vi "Configure Bursted Generation.vi"(0 "RFSG handle":refnum<k15>, 5 "Waveform":T1={"Waveform Name"="Wfm", "Waveform"={"x0"=0.0, "dx"=0.0, "y"=[]}, "Signal Bandwidth (Hz)"=0.0, "PAPR (dB)"=0.0, "Burst Length (s)"=0.0, "Sample Rate"=0.0, "Burst Start Locations"=[], "Burst Stop Locations"=[], "Idle Duration Present?"=FALSE, "Runtime Scaling"=0.0, "Script"=""} {"Runtime Scaling" format="%#_6p"; "Sample Rate" format="%#_6p"; "Burst Length (s)" format="%#_6p"; "PAPR (dB)" format="%.2f"; "Signal Bandwidth (Hz)" format="%#_6p"; "Waveform"."y" format="%.2f"; "Waveform"."dx" format="%^.2e"; "Waveform"."x0" format="%^.2e"}, 7 "Waveform Timing Configuration":T4={"Duty Cycle (%)"=50.0, "Pre-Burst Time (s)"=1e-06, "Post-Burst Time (s)"=1e-06, "Burst Start Trigger Export"="PXI_Trig0"} {"Post-Burst Time (s)" format="%#_6p"; "Pre-Burst Time (s)" format="%#_6p"; "Duty Cycle (%)" min=1.0 max=100.0 step=1.0 format="%#_2d%%"}, 9 "PAEN Configuration":T2={"PAEN Mode"=enum."Dynamic", "PA Enable Trigger Export Terminal"="PFI0", "PA Enable Trigger Mode"=23001, "Command Enable Time (s)"=0.0, "Command Disable Time (s)"=0.0} {"PA Enable Trigger Mode" items=["Pulse"=23000, "Toggle"=23001]; "Command Disable Time (s)" format="%#_6p"; "Command Enable Time (s)" format="%#_6p"}, 11 "error in":errorcluster) -> (4 "RFSG handle out":refnum<k15>, 6 "Waveform out":T1={"Waveform Name"="Wfm", "Waveform"={"x0"=0.0, "dx"=0.0, "y"=[]}, "Signal Bandwidth (Hz)"=0.0, "PAPR (dB)"=0.0, "Burst Length (s)"=0.0, "Sample Rate"=0.0, "Burst Start Locations"=[], "Burst Stop Locations"=[], "Idle Duration Present?"=FALSE, "Runtime Scaling"=0.0, "Script"=""} {"Runtime Scaling" format="%#_6p"; "Sample Rate" format="%#_6p"; "Burst Length (s)" format="%#_6p"; "PAPR (dB)" format="%.2f"; "Signal Bandwidth (Hz)" format="%#_6p"; "Waveform"."y" format="%.2f"; "Waveform"."dx" format="%^.2e"; "Waveform"."x0" format="%^.2e"}, 8 "Generation Period (s)":dbl format="%#_6p", 15 "error out":errorcluster)   [LabVIEW 2016, in "SG.lvlib"]
uses:
  SG.lvlib
  Typedefs/Waveform.ctl
  Typedefs/Waveform Timing Configuration.ctl
  <instrlib>/niRFSG/niRFSG.llb/niRFSG Exported Signal Destinations.ctl
  Typedefs/PAEN Configuration.ctl
  <instrlib>/niRFSG/niRFSG.llb/niRFSG Signal Names.ctl
  <instrlib>/niRFSG/niRFSG.llb/niRFSG Signal Identifiers.ctl
  <instrlib>/niRFSG/niRFSG.llb/niRFSG Script Trigger IDs.ctl
  <instrlib>/niRFSG/niRFSG.llb/niRFSG Configure Script Trigger Software.vi
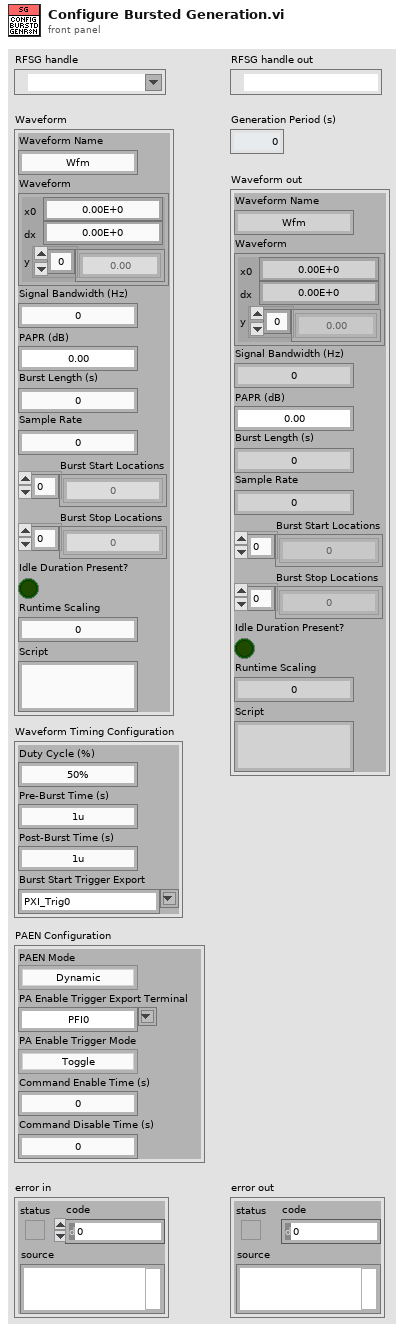
[diagram p1: front panel]
types:
  T1 = typedef "SG.lvlib/Waveform.ctl" = cluster{"Waveform Name":string, "Waveform":cluster{"x0":dbl, "dx":dbl, "y":csg[]}, "Signal Bandwidth (Hz)":dbl, "PAPR (dB)":dbl, "Burst Length (s)":dbl, "Sample Rate":dbl, "Burst Start Locations":i32[], "Burst Stop Locations":i32[], "Idle Duration Present?":bool, "Runtime Scaling":dbl, "Script":string}
  T2 = typedef "SG.lvlib/PAEN Configuration.ctl" = cluster{"PAEN Mode":enum16{"Disabled", "Static", "Dynamic"}, "PA Enable Trigger Export Terminal":T3, "PA Enable Trigger Mode":i32, "Command Enable Time (s)":dbl, "Command Disable Time (s)":dbl}
  T3 = typedef "niRFSG Exported Signal Destinations.ctl" = string
  T4 = typedef "SG.lvlib/Waveform Timing Configuration.ctl" = cluster{"Duty Cycle (%)":dbl, "Pre-Burst Time (s)":dbl, "Post-Burst Time (s)":dbl, "Burst Start Trigger Export":T3}
  T5 = typedef "niRFSG Script Trigger IDs.ctl" = string
  T6 = typedef "niRFSG Signal Identifiers.ctl" = string
  T7 = typedef "niRFSG Signal Names.ctl" = i32
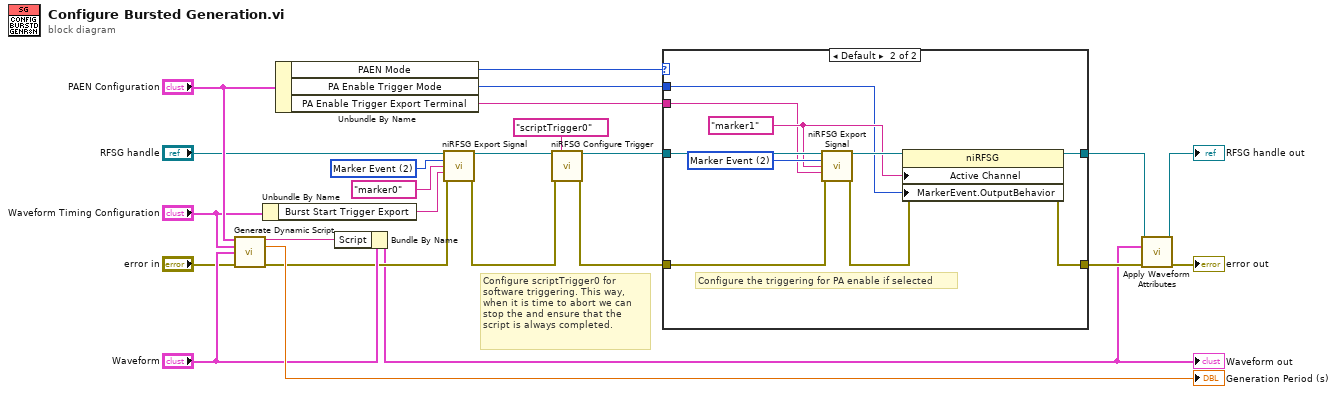
[diagram p0: block diagram]
diagram:
  w17 = T7 2 items=["Start Trigger", "Script Trigger", "Marker Event", "Ref Clock", "Started Event", "Done Event", "Configuration List Step Trigger", "Configuration Settled Event"] ("signal")
  # "Configure scriptTrigger0 for software triggering. This way, when it is time to abort we can stop the and ensure that the script is always completed."
  n1 = call "Generate Dynamic Script.vi"("PAEN Config"="PAEN Configuration", "Waveform Timing Configuration"="Waveform Timing Configuration", "Waveform"="Waveform", "error in (no error)"="error in") -> ("Script"=w8:string, "Generation Period (s)"=→"Generation Period (s)":dbl, "error out"=w6:errorcluster)  [unwired: 9 in]
  n2 = Unbundle By Name("Waveform Timing Configuration") -> ("Burst Start Trigger Export"=w14:T3)
  n3 = Unbundle By Name("PAEN Configuration") -> ("PAEN Mode"=w21:enum16{"Disabled", "Static", "Dynamic"}, "PA Enable Trigger Mode"=w20:i32, "PA Enable Trigger Export Terminal"=w18:T3)
  n4 = Bundle By Name(cluster="Waveform", "Script"=w8) -> (w1:T1)
  "Waveform out" <- w1
  n5 = call <instrlib>:"niRFSG Export Signal.vi"("instrument handle"="RFSG handle", "signal"=w17, "signal identifier"=T6 "marker0", "output terminal"=w14, "error in"=w6) -> ("instrument handle out"=w12:refnum<k15>, "error out"=w11:errorcluster)  [unwired: 9 in]
  n6 = call-poly <instrlib>:"niRFSG Configure Trigger.vi"("instrument handle"=w12, "trigger id"=T5 "scriptTrigger0", "error in"=w11) -> ("instrument handle out"=w9:refnum<k15>, "error out"=w10:errorcluster)  [unwired: 11 in]
  n7 = case "Configure the triggering for PA enable if selected" shown="Default" w21 {
    tunnel: [w26 w27] -> w3
    tunnel: w10 -> [w26 w33]
    tunnel: [w25 w28] -> w4
    tunnel: w9 -> [w25 w36]
    tunnel: w20 -> [_ w30]
    tunnel: w18 -> [_ w29]
    frame "Disabled" {
    }
    frame Default {
      w31 = T6 "marker1" ("signal identifier")
      w34 = T7 2 items=["Start Trigger", "Script Trigger", "Marker Event", "Ref Clock", "Started Event", "Done Event", "Configuration List Step Trigger", "Configuration Settled Event"] ("signal")
      # "Configure the triggering for PA enable if selected"
      n8 = call <instrlib>:"niRFSG Export Signal.vi"("instrument handle"=w36, "signal"=w34, "signal identifier"=w31, "output terminal"=w29, "error in"=w33) -> ("instrument handle out"=w35:refnum<k15>, "error out"=w32:errorcluster)  [unwired: 9 in]
      n9 = property class="niRFSG"(reference=w35, error in=w32, "Active Channel"=w31, "MarkerEvent.OutputBehavior"=w30) -> (reference out=w28:refnum<k15>, error out=w27:errorcluster)
    }
  }
  n10 = call "Apply Waveform Attributes.vi"("RFSG Session In"=w4, "Waveform"=w1, "error in (no error)"=w3) -> ("RFSG Session Out"=→"RFSG handle out":refnum<k15>, "error out"=→"error out":errorcluster)  [unwired: 11 in]
